vi "q4 parking charges.vi"() -> ()   [LabVIEW 2025]
panel:
  out "PRICE":dbl
  in  "HOURS":dbl
  in  "ON IS FOUR WHEELER":bool
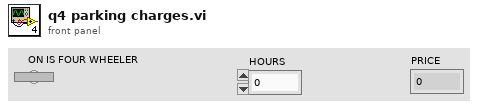
[diagram p1: front panel]
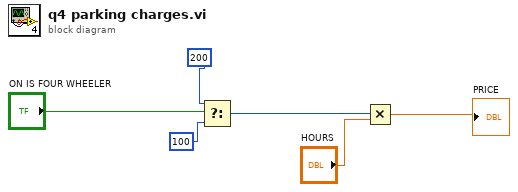
[diagram p0: block diagram]
diagram:
  n1 = Select(t=200, s="ON IS FOUR WHEELER", f=100) -> (s? t:f=w3:i32)
  n2 = Multiply(x=w3, y="HOURS") -> (x*y=→"PRICE":dbl)
